vi "ex_AddHeaderElementToArray.vi"(8 "error in (no error)":errorcluster, 9 "string":string, 10 "name":string, 11 "string array in":string[][](array[string])) -> (0 "error out":errorcluster, 3 "string array out":string[][](array[string]))   [LabVIEW 2020]
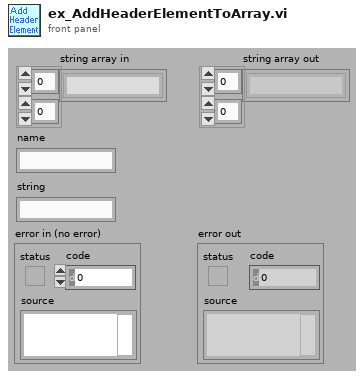
[diagram p1: front panel]
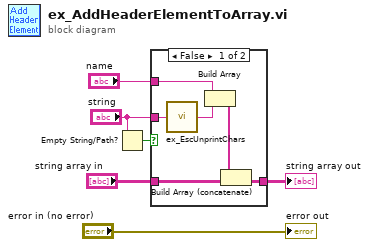
[diagram p0: block diagram]
diagram:
  n1 = Empty String/Path?(string/path="string") -> (empty?=w5:bool)
  n2 = case shown="False" w5 {
    tunnel: "string" -> [w11 _]
    tunnel: "name" -> [w12 _]
    tunnel: "string array in" -> [w10 w13]
    tunnel: [w8 w13] -> w1
    frame False {
      n3 = call "ex_EscUnprintChars.vi"("input"=w11) -> ("output"=w7:string)
      n4 = Build Array(w12, w7) -> (w9:string[])
      n5 = Build Array (concatenate)(w9, w10) -> (w8:string[][])
    }
    frame True {
    }
  }
  "string array out" <- w1
  "error out" <- "error in (no error)"
